vi "Basic Hardware Loop.vi"() -> ()   [LabVIEW 2018]
doc: "Creates a basic loop structure. It is the user's responsibility to fill in the contents of the loop. However, this template includes the initial hardware configuration and contains a Control and Simulation Loop preconfigured for a 500 Hz sample time."
uses:
  <vilib>/Simulation/Scripting/Companion Diagram/SimConfigNode/SimParams.ctl
  <vilib>/Simulation/Scripting/Companion Diagram/SimConfigNode/_simSolvers.ctl
  <vilib>/Simulation/Implementation/Shared/SIMSCR Execution Mode.ctl
  <vilib>/Platform/TimedLoop/XDataNode/timing_clust.ctl
  <vilib>/Platform/TimedLoop/XDataNode/nitl_modes.ctl
  <vilib>/Platform/TimedLoop/XDataNode/wakeup.ctl
  <vilib>/Simulation/Param Hierarchy/Typedefs/SIMPH Param Control Actions.ctl
  <vilib>/Simulation/Implementation/Shared/NILVSim_ParamChanged.vi
  <vilib>/Simulation/Implementation/Shared/NILVSim_FinishedLate.vi
  <vilib>/Simulation/Implementation/Shared/NILVSIM_BeginStep.vi
  <vilib>/Simulation/Utility/Implementation/SIM Halt.vi
  <vilib>/Simulation/DataSources/Implementation/NILVSim Signal Generator.llb/SIM Signal Generator (scalar).vi
  <vilib>/Simulation/SignalArithmetic/Implementation/NILVSim Gain.llb/SIM Gain (scalar).vi
  <vilib>/Simulation/ContinuousLinear/Implementation/NILVSim Transfer Function Direct.llb/SIM Transfer Function Direct (SISO).vi
  <vilib>/Simulation/SignalArithmetic/Implementation/NILVSim Gain.llb/SIM Gain (dot product).vi
  <vilib>/Simulation/Implementation/Shared/NILVSim_Manager.vi
  <vilib>/Utility/error.llb/Clear Errors.vi
  <vilib>/Simulation/Implementation/Shared/NILVSim_FinalizeModel.vi
  <vilib>/Simulation/Implementation/Shared/SIM Unbundle Sim Info.vi
  <vilib>/Simulation/Implementation/Shared/SIMSH Read Queue.vi
  <vilib>/Simulation/Implementation/Shared/NILVSim_Initialize.vi
  <vilib>/Simulation/Utility/Implementation/NILVSim Get Time and IsAcceptedStep.vi
  <vilib>/Simulation/Implementation/Shared/NILVSim_GetModelError.vi
  <vilib>/Simulation/Implementation/Shared/SIM Bundle Sim Info.vi
  <vilib>/Simulation/Scripting/Companion Diagram/SimConfigNode/SimDog.xnode
  <vilib>/Quanser/Rapid Control Prototyping Toolkit/hardware/HIL Immediate IO/_TypeSpecific/CL HIL Read Encoder (Vector).vi
  <vilib>/Quanser/Rapid Control Prototyping Toolkit/hardware/HIL Immediate IO/CL HIL Read.vi
  <vilib>/Quanser/Rapid Control Prototyping Toolkit/hardware/HIL Immediate IO/_TypeSpecific/CL HIL Write Analog (Scalar).vi
  <vilib>/Quanser/Rapid Control Prototyping Toolkit/hardware/HIL Immediate IO/CL HIL Write.vi
  Downloads/QUBE ROTPEN Encoders to Angles.vi
  <vilib>/Platform/TimedLoop/XDataNode/XDataNode.xnode
  <vilib>/Simulation/Implementation/XNodeFramework/SimXNode/SimX.xnode
  <vilib>/Platform/TimedLoop/XDataNode/XDNodeRunTimeDep.lvlib
  <vilib>/Simulation/Implementation/Shared/NI_SIM_Implementation.lvlib
panel:
  out "DC motor (volt)":dbl(graph)
  out "Encoder Arm (deg)":cluster{"output":dbl, "output":dbl}(graph)
  out "Rotary Pendulum (deg)":dbl(graph)
  in  "Gain, K":dbl[](array[numeric])=[-1.0, 30.0, -1.25, 3.0]
  in  "Freq (Hz)":dbl=0.12500000000000003 min=0.005 max=1.0 step=0.005
  in  "Amp (deg)":dbl min=0.0 max=90.0 step=5.0
  out "Error":errorcluster
  in  "Stop Button":bool
  # "See the block diagram for instructions\non using this basic hardware template."
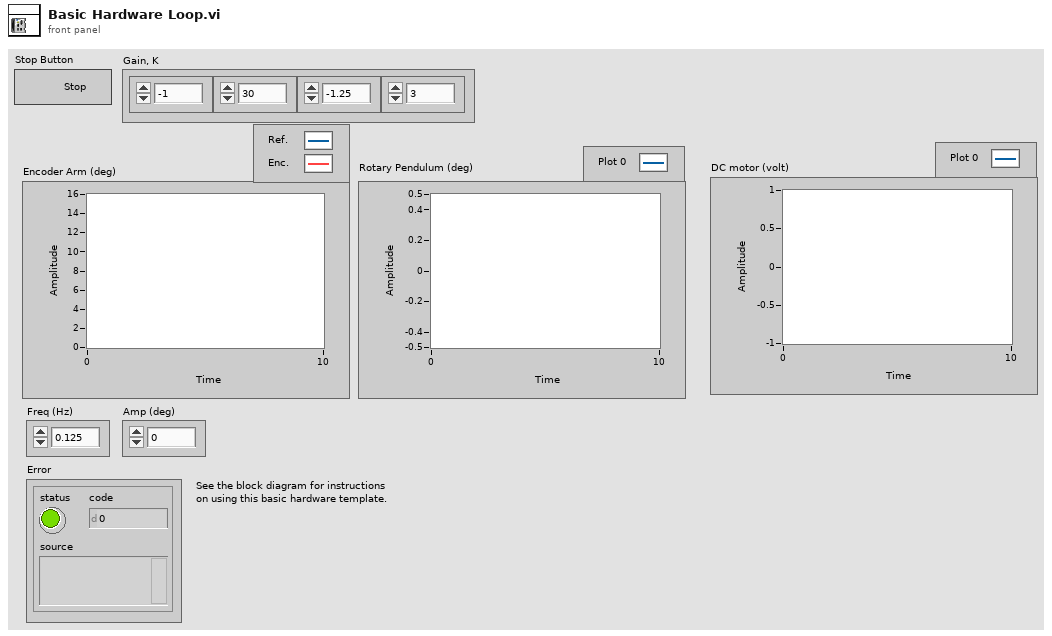
[diagram p1: front panel]
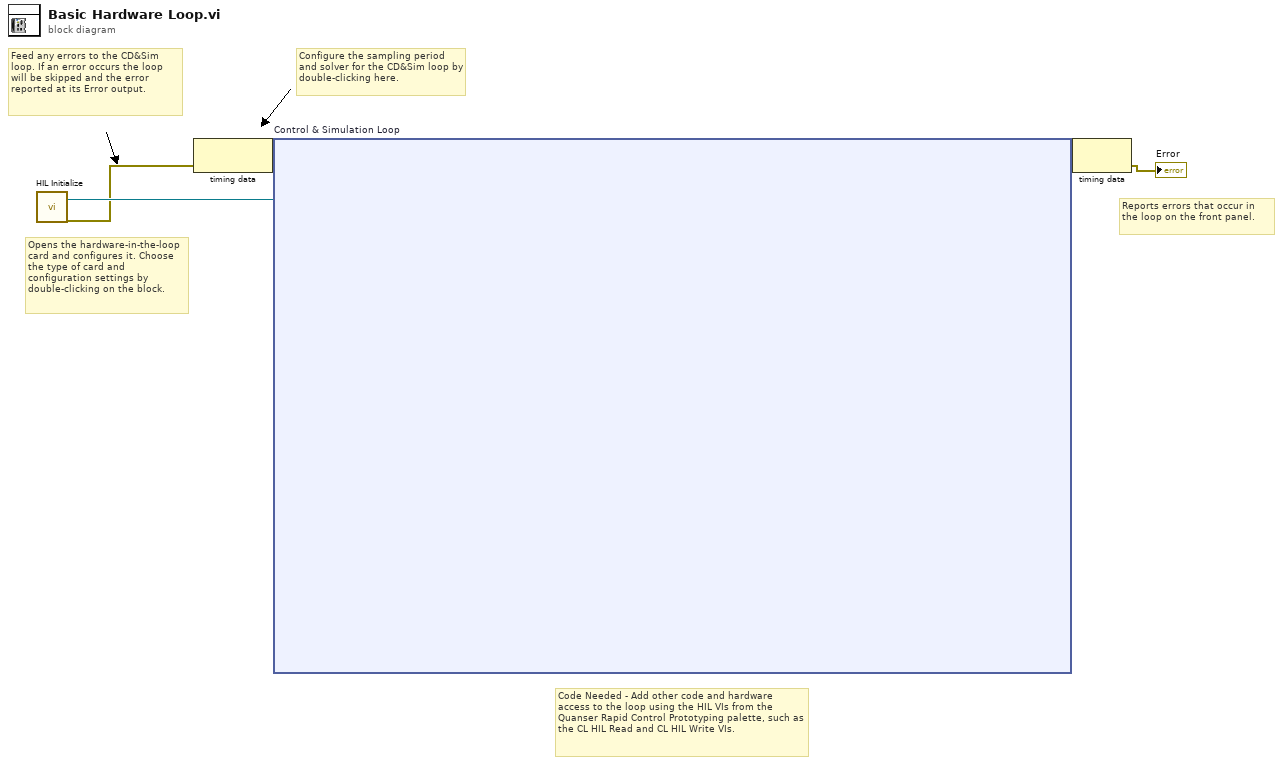
[diagram p0: block diagram]
diagram:
  # "Code Needed - Add other code and hardware access to the loop using the HIL VIs from the Quanser Rapid Control Prototyping palette, such as the CL HIL Read and CL HIL Write VIs."
  # "Configure the sampling period  and solver for the CD&Sim loop by double-clicking here."
  # "Reports errors that occur in the loop on the front panel."
  # "Feed any errors to the CD&Sim loop. If an error occurs the loop will be skipped and the error reported at its Error output."
  # "Opens the hardware-in-the-loop card and configures it. Choose the type of card and configuration settings by double-clicking on the block."
  n1 = call "HIL Initialize"() -> ("board out"=w2:refnum<class "HIL Board.lvclass">, "error out"=w1:errorcluster)  [unwired: 14 in]
  n2 = node-c288(w1) -> (w5:variant)
  n3 = node-c254 "Control & Simulation Loop"(w5, w2) -> (w4:variant)
  n4 = node-c288(w4) -> (→"Error":errorcluster)
